vi "SR.vi"() -> ()   [LabVIEW 2018]
panel:
  in  "stop":bool
  out "Z0":bool
  out "Z1":bool
  out "Q0":bool
  out "Q1":bool
  in  "Y":bool
  in  "X":bool
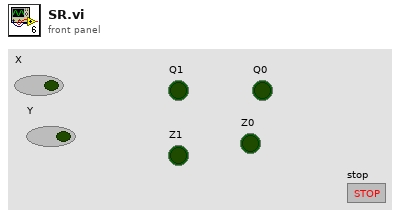
[diagram p1: front panel]
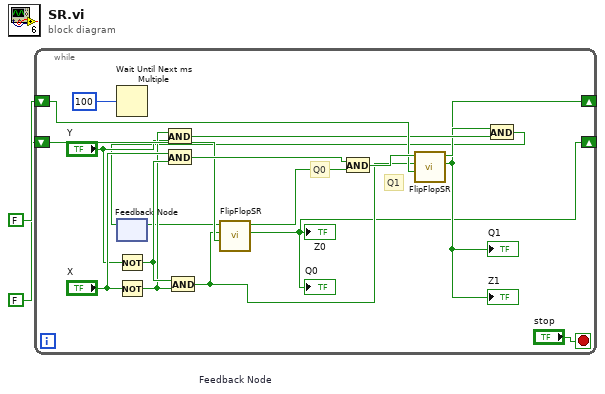
[diagram p0: block diagram]
diagram:
  n1 = while {
    shift-right: [w3] -> _
    shift-left: FALSE -> [w15]
    shift-right: [w4] -> _
    shift-left: FALSE -> [w16]
    stop <- "stop" stop-if-true
    # "Q0"
    # "Q1"
    n2 = Wait Until Next ms Multiple(millisecond multiple=u32 100) -> ()  [unwired: 1 out]
    n3 = feedback #1 "Feedback Node"() -> (w8:bool)  [unwired: 1 in]
    n4 = Not(x="Y") -> (.not. x?=w18:bool)
    n5 = Not(x="X") -> (.not. x?=w14:bool)
    n6 = And(x=w14, y="Y") -> (x .and. y?=w11:bool)
    n7 = And(x="X", y=w18) -> (x .and. y?=w20:bool)
    n8 = And(x=w18, y=w14) -> (x .and. y?=w7:bool)
    n9 = call "FlipFlopSR.vi"("Q"=w15, "Reset"=w7, "Set"=w8) -> ("Q*"=w3:bool, "QN*"=w12:bool)  [unwired: 7 in]
    "Q0" <- w3
    "Z0" <- w3
    n10 = And(x=w20, y=w12) -> (x .and. y?=w19:bool)
    n11 = call "FlipFlopSR.vi"("Q"=w16, "Reset"=w7, "Set"=w19) -> ("Q*"=w4:bool, "QN*"=w10:bool)  [unwired: 7 in]
    "Q1" <- w4
    "Z1" <- w4
    n12 = And(x=w10, y=w11) -> (x .and. y?=w9:bool)
    n13 = feedback-in #1(w9) -> ()
  }
